vi "iexpress - Create Self-Extracting Archive.vi"(4 "License Agreement .txt (none)":path, 5 "Prompt (none)":string, 6 "Finish Message (none)":string, 7 "Title (none)":string, 8 "error in (no error)":errorcluster, 9 "Launch on Extract":path, 10 "Target Archive (.exe)":path, 11 "File or Folder Path":path) -> (0 "error out":errorcluster, 3 "Path to Archive":path)   [LabVIEW 2011]
uses:
  OpenG EXT/file/file.llb/File Exists - Scalar__ogtk.vi
  OpenG EXT/file/file.llb/Append Path to Root if Relative - Scalar__ogtk.vi
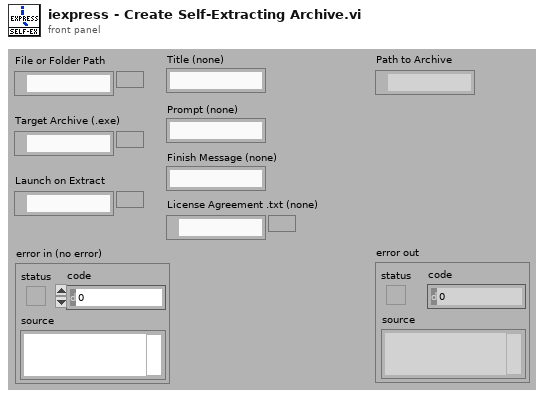
[diagram p1: front panel]
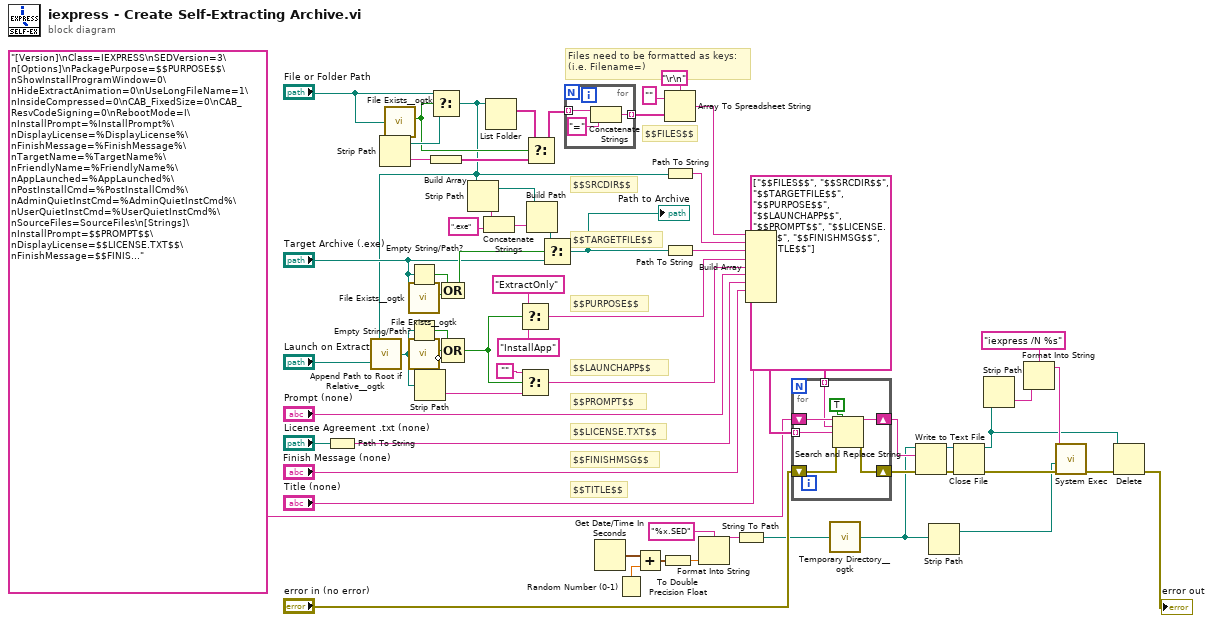
[diagram p0: block diagram]
diagram:
  # "$$TITLE$$"
  # "$$FINISHMSG$$"
  # "$$LICENSE.TXT$$"
  # "$$PROMPT$$"
  # "$$FILES$$"
  # "$$LAUNCHAPP$$"
  # "$$TARGETFILE$$"
  # "$$SRCDIR$$"
  # "$$PURPOSE$$"
  # "Files need to be formatted as keys:\n(i.e. Filename=)"
  n1 = Path To String(path="License Agreement .txt (none)") -> (string=w3:string)
  n2 = Strip Path(path="File or Folder Path") -> (stripped path=w63:path, name=w48:string)
  n3 = call-poly "File Exists__ogtk.vi"("file path"="File or Folder Path") -> ("is directory"=w45:bool)  [unwired: 6 in, 1 out]
  n4 = Empty String/Path?(string/path="Target Archive (.exe)") -> (empty?=w55:bool)
  n5 = call-poly "File Exists__ogtk.vi"("file path"="Target Archive (.exe)") -> ("is directory"=w56:bool)  [unwired: 6 in, 1 out]
  n6 = Select(t="File or Folder Path", s=w45, f=w63) -> (s? t:f=w8:path)
  n7 = call-poly "Append Path to Root if Relative__ogtk.vi"("Absolute or Relative Path"="Launch on Extract", "Root Path"=w8) -> ("Absolute or Appended Path"=w11:path)
  n8 = Empty String/Path?(string/path=w11) -> (empty?=w62:bool)
  n9 = call-poly "File Exists__ogtk.vi"("file path"=w11) -> ("is directory"=w61:bool, "exists"=w60:bool)  [unwired: 6 in]
  n10 = Strip Path(path=w11) -> (name=w58:string)  [unwired: 1 out]
  n11 = Build Array(w48) -> (w46:string[])
  n12 = Compound Arithmetic op=OR(w55, w56) -> (w50:bool)
  n13 = Compound Arithmetic op=OR(w62, w61, invert w60) -> (w57:bool)
  n14 = Strip Path(path=w8) -> (stripped path=w12:path, name=w54:string)
  n15 = Concatenate Strings(w54, ".exe") -> (w52:string)
  n16 = List Folder(path=w8) -> (filenames=w47:string[])  [unwired: 1 in, 5 out]
  n17 = Select(t="ExtractOnly", s=w57, f="InstallApp") -> (s? t:f=w38:string)
  n18 = Select(t="", s=w57, f=w58) -> (s? t:f=w37:string)
  n19 = Select(t=w47, s=w45, f=w46) -> (s? t:f=w44:string[])
  n20 = Build Path(base path=w12, name or relative path=w52) -> (appended path=w51:path)
  n21 = Select(t=w51, s=w50, f="Target Archive (.exe)") -> (s? t:f=w32:path)
  "Path to Archive" <- w32
  n22 = for {
    tunnel: w44 -> [w68] mode=indexing
    tunnel: [w66] -> w43 mode=indexing
    n23 = Concatenate Strings(w68, "=") -> (w66:string)
  }
  n24 = Get Date/Time In Seconds() -> (seconds since 1Jan1904=w30:timestamp)
  n25 = Random Number (0-1)() -> (number: 0 to 1=w31:dbl)
  n26 = Add(x=w30, y=w31) -> (x+y=w28:timestamp)
  n27 = To Double Precision Float(number=w28) -> (double precision float=w27:dbl)
  n28 = Array To Spreadsheet String(delimiter (Tab)="\r\n", array=w43, 3:"") -> (spreadsheet string=w41:string)
  n29 = Path To String(path=w8) -> (string=w40:string)
  n30 = Path To String(path=w32) -> (string=w39:string)
  n31 = Format Into String(format string="%x.SED", w27) -> (resulting string=w26:string)  [unwired: 2 in, 1 out]
  n32 = String To Path(string=w26) -> (path=w25:path)
  n33 = Build Array(w41, w40, w39, w38, w37, "Prompt (none)", w3, "Finish Message (none)", "Title (none)") -> (w36:string[])
  n34 = for {
    tunnel: w36 -> [w73] mode=indexing
    shift-right: [w72] -> w23
    shift-left: "[Version]\nClass=IEXPRESS\nSEDVersion=3\n[Options]\nPackagePurpose=$$PURPOSE$$\nShowInstallProgramWindow=0\nHideExtractAnimation=0\nUseLongFileName=1\nInsideCompressed=0\nCAB_FixedSize=0\nCAB_ResvCodeSigning=0\nRebootMode=I\nInstallPrompt=%InstallPrompt%\nDisplayLicense=%DisplayLicense%\nFinishMessage=%FinishMessage%\nTargetName=%TargetName%\nFriendlyName=%FriendlyName%\nAppLaunched=%AppLaunched%\nPostInstallCmd=%PostInstallCmd%\nAdminQuietInstCmd=%AdminQuietInstCmd%\nUserQuietInstCmd=%UserQuietInstCmd%\nSourceFiles=SourceFiles\n[Strings]\nInstallPrompt=$$PROMPT$$\nDisplayLicense=$$LICENSE.TXT$$\nFinishMessage=$$FINISHMSG$$\nTargetName=$$TARGETFILE$$\nFriendlyName=$$TITLE$$\nAppLaunched=$$LAUNCHAPP$$\nPostInstallCmd=<None>\nAdminQuietInstCmd=\nUserQuietInstCmd=\n[SourceFiles]\nSourceFiles0=$$SRCDIR$$\n[SourceFiles0]\n$$FILES$$" -> [w75]
    tunnel: string[] ["$$FILES$$", "$$SRCDIR$$", "$$TARGETFILE$$", "$$PURPOSE$$", "$$LAUNCHAPP$$", "$$PROMPT$$", "$$LICENSE.TXT$$", "$$FINISHMSG$$", "$$TITLE$$"] -> [w74] mode=indexing
    shift-right: [w70] -> w24
    shift-left: "error in (no error)" -> [w71]
    n35 = Search and Replace String(replace all?=TRUE ("replace all? (F)"), input string=w75, search string=w74, replace string=w73, error in=w71) -> (result string=w72:string, error out=w70:errorcluster)  [unwired: 5 out]
  }
  n36 = call "Temporary Directory__ogtk.vi"("Relative path (.)"=w25) -> ("Temporary Directory (+ Relative)"=w17:path)
  n37 = Write to Text File(file (use dialog)=w17, text=w23, error in=w24) -> (refnum out=w21:refnum<file>, error out=w22:errorcluster)  [unwired: 2 out]
  n38 = Strip Path(path=w17) -> (stripped path=w16:path)  [unwired: 1 out]
  n39 = Close File(refnum=w21, error in=w22) -> (path=w7:path, error out=w18:errorcluster)
  n40 = Strip Path(path=w7) -> (name=w6:string)  [unwired: 1 out]
  n41 = Format Into String(format string="iexpress /N %s" ("command line"), w6) -> (resulting string=w19:string)  [unwired: 2 in, 1 out]
  n42 = call <vilib>:"System Exec.vi"("error in (no error)"=w18, "working directory"=w16, "command line"=w19) -> ("error out"=w15:errorcluster)  [unwired: 3 in, 5 out]
  n43 = Delete(path (use dialog)=w7, error in=w15) -> (error out=→"error out":errorcluster)  [unwired: 5 out]
